vi "Write Switch Heater (No Objects).vi"(8 "error in (no error)":errorcluster, 10 "Turn SH On?":bool, 11 "Cluster In":T4={"Field"=0.0, "Rate"=0.0, "Status"={"Sweeping"=FALSE, "Clamped"=FALSE, "Hold"=FALSE, "At Rest"=FALSE, "Quench"=FALSE, "Persistent Mode"=FALSE, "Switch Heater"=FALSE}, "ILM Shut Down?"=FALSE, "IO Info"={"Address"={"Com Port"=1, "ISOBUS Address"=2, "GPIB Address"=24, "Communication"=enum."ISOBUS"}, "Version"=enum."IPS"}, "IO Info (Level Meter)"={"Address"={"Com Port"=1, "ISOBUS Address"=5, "GPIB Address"=24, "Communication"=enum."ISOBUS"}, "ILM Name"="", "Display Channel"=[]}, "Training?"=FALSE, "Training Field and Speed Cluster"={"Training Field"=[0.0, 4.108, 5.78, 8.001], "Training Speed"=[0.0057, 0.0022833333333333334, 0.0011333333333333334, 0.0011333333333333334]}}) -> (0 "error out":errorcluster, 3 "Cluster Out":T4={"Field"=0.0, "Rate"=0.0, "Status"={"Sweeping"=FALSE, "Clamped"=FALSE, "Hold"=FALSE, "At Rest"=FALSE, "Quench"=FALSE, "Persistent Mode"=FALSE, "Switch Heater"=FALSE}, "ILM Shut Down?"=FALSE, "IO Info"={"Address"={"Com Port"=1, "ISOBUS Address"=2, "GPIB Address"=24, "Communication"=enum."ISOBUS"}, "Version"=enum."IPS"}, "IO Info (Level Meter)"={"Address"={"Com Port"=1, "ISOBUS Address"=5, "GPIB Address"=24, "Communication"=enum."ISOBUS"}, "ILM Name"="", "Display Channel"=[]}, "Training?"=FALSE, "Training Field and Speed Cluster"={"Training Field"=[0.0, 4.108, 5.78, 8.001], "Training Speed"=[0.0057, 0.0022833333333333334, 0.0011333333333333334, 0.0011333333333333334]}})   [LabVIEW 2012]
uses:
  Magnet status.ctl
  Oxford/PSSUBS.LLB/PSIO.ctl
  Oxford/BUSGEN.LLB/OxfordAddress.ctl
  Switch Heater Status.ctl
  Power Supply.lvclass
panel:
  out "true interrupt":bool
  in  "interrupt":bool
  out "done":bool
  out "busybar":bool[](array[boolean])
  out "time":string
  out "display":string
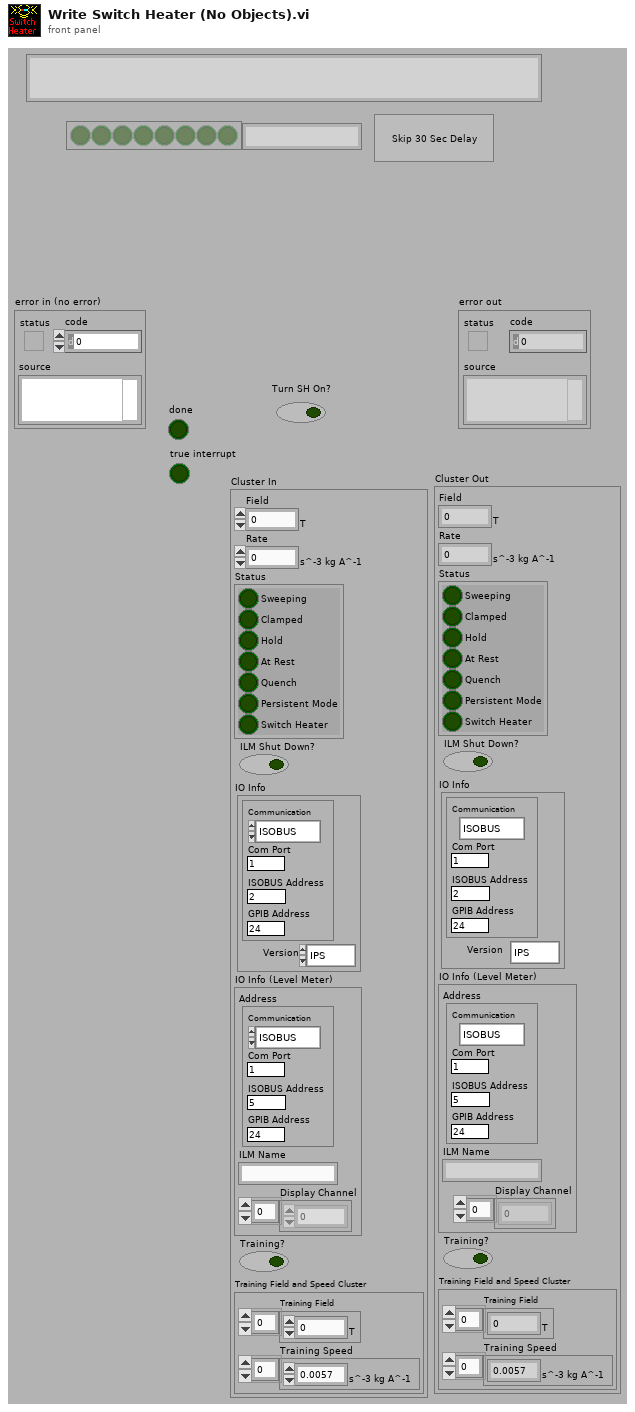
[diagram p1: front panel]
types:
  T1 = typedef "Power Supply.lvclass/Magnet status.ctl" = cluster{"Sweeping":bool, "Clamped":bool, "Hold":bool, "At Rest":bool, "Quench":bool, "Persistent Mode":bool, "Switch Heater":bool}
  T2 = typedef "PSIO.ctl" = cluster{"Address":T3, "Version":enum16{"PS", "IPS"}}
  T3 = typedef "OxfordAddress.ctl" = cluster{"Com Port":i32, "ISOBUS Address":i32, "GPIB Address":i16, "Communication":enum16{"RS232", "ISOBUS", "GPIB", "Gateway"}}
  T4 = cluster{"Field":dbl[unit], "Rate":dbl[unit], "Status":T1, "ILM Shut Down?":bool, "IO Info":T2, "IO Info (Level Meter)":cluster{"Address":T3, "ILM Name":string, "Display Channel":i32[]}, "Training?":bool, "Training Field and Speed Cluster":cluster{"Training Field":dbl[unit][], "Training Speed":dbl[unit][]}}
  T5 = typedef "Power Supply.lvclass/Switch Heater Status.ctl" = enum16{"Off (at zero)", "On", "Off (at field)", "Other"}
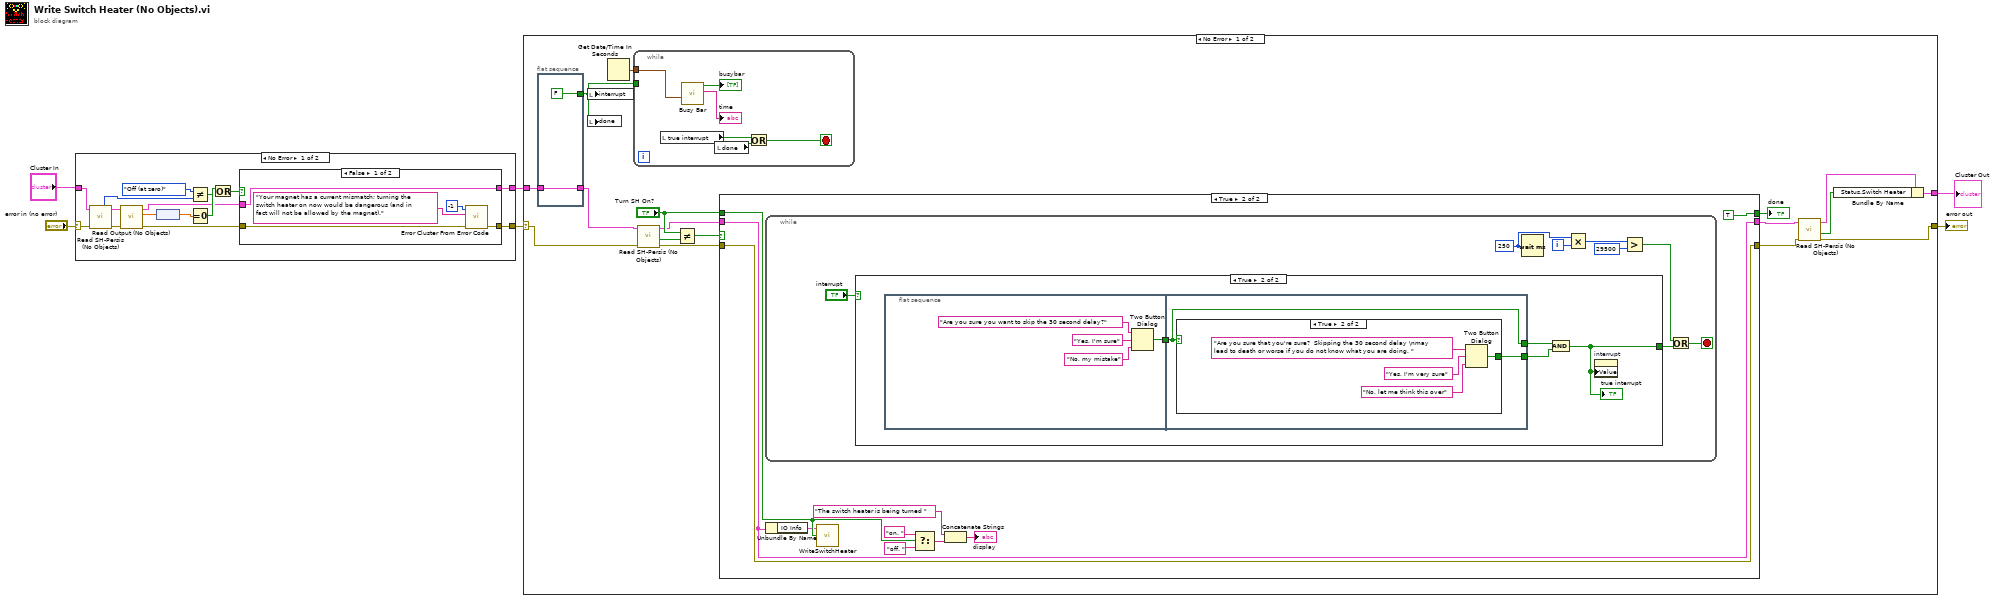
[diagram p0: block diagram]
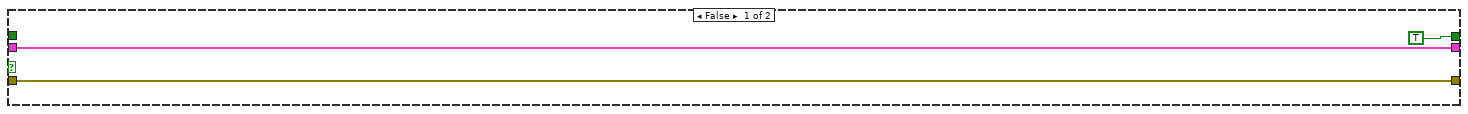
[diagram p4: hidden frame]
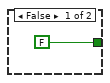
[diagram p5: hidden frame]
diagram:
  n1 = case shown="No Error" "error in (no error)" {
    selector: "error in (no error)" -> [w12 w29]
    tunnel: [w14 w30] -> w5
    tunnel: [w13 w29] -> w4
    tunnel: "Cluster In" -> [w8 w30]
    frame No Error {
      n2 = call "Read SH-Persis (No Objects).vi"("error in (no error)"=w12, "Cluster In"=w8) -> ("error out"=w17:errorcluster, "Cluster Out"=w7:T4, "SHstatus"=w11:T5)  [unwired: 4 in, 3 out]
      n3 = call "Read Output (No Objects).vi"("error in (no error)"=w17, "Cluster In"=w7) -> ("error out"=w18:errorcluster, "Field"=w19:dbl[unit], "Cluster Out"=w16:T4)  [unwired: 6 in, 1 out]
      n4 = node(w19) -> (w15:dbl)
      n5 = Not Equal?(x=Switch_Heater_Status."Off (at zero)", y=w11) -> (x != y?=w9:bool)
      n6 = Equal To 0?(x=w15) -> (x = 0?=w21:bool)
      n7 = Or(x=w21, y=w9) -> (x .or. y?=w20:bool)
      n8 = case shown="False" w20 {
        tunnel: w18 -> [w25 w28]
        tunnel: w16 -> [w26 w27]
        tunnel: [w26 w27] -> w14
        tunnel: [w24 w28] -> w13
        frame False {
          n9 = call <vilib>:"Error Cluster From Error Code.vi"("error in (no error)"=w25, "error message (\"\")"="Your magnet has a current mismatch; turning the switch heater on now would be dangerous (and in fact will not be allowed by the magnet).", "error code (0)"=-1) -> ("error out"=w24:errorcluster)  [unwired: 6 in]
        }
        frame True {
        }
      }
    }
    frame Error {
    }
  }
  n10 = case shown="No Error" w4 {
    selector: w4 -> [w44 w92]
    tunnel: w5 -> [w47 w93]
    tunnel: [w46 w93] -> w1
    tunnel: [w45 w92] -> w6
    frame No Error {
      n11 = flat-sequence {
        tunnel: w47 -> [w91]
        tunnel: [w91] -> w32
        tunnel: [FALSE] -> w33
        frame #0 {
        }
      }
      n12 = local write "interrupt"(w33) -> ()
      n13 = local write "done"(w33) -> ()
      n14 = Get Date/Time In Seconds() -> (seconds since 1Jan1904=w43:timestamp)
      n15 = while {
        tunnel: w43 -> [w84]
        tunnel: w33 -> [_]
        stop <- w87 stop-if-true
        n16 = local read "true interrupt"() -> (w85:bool)
        n17 = call "Busy Bar.vi"("basetime"=w84) -> ("Time"=→"time":string, "Busy Bar"=→"busybar":bool[])  [unwired: 1 in, 8 out]
        n18 = local read "done"() -> (w86:bool)
        n19 = Or(x=w85, y=w86) -> (x .or. y?=w87:bool)
      }
      n20 = call "Read SH-Persis (No Objects).vi"("error in (no error)"=w44, "Cluster In"=w32) -> ("error out"=w37:errorcluster, "SHon?"=w39:bool, "Cluster Out"=w38:T4)  [unwired: 4 in, 3 out]
      n21 = Not Equal?(x="Turn SH On?", y=w39) -> (x != y?=w41:bool)
      n22 = case shown="True" w41 {
        tunnel: "Turn SH On?" -> [_ w60]
        tunnel: [w50 w54] -> w31
        tunnel: w38 -> [w50 w54]
        tunnel: w37 -> [w49 w52]
        tunnel: [w49 w52] -> w42
        tunnel: [TRUE TRUE] -> w36
        frame False {
        }
        frame True {
          n23 = while {
            i -> [w67]
            stop <- w68 stop-if-true
            w66 = 250
            n24 = case shown="True" "interrupt" {
              tunnel: [FALSE w70] -> w61
              frame False {
              }
              frame True {
                n25 = flat-sequence {
                  tunnel: [w74] -> w71
                  tunnel: [w78] -> w73
                  tunnel: w71 -> [w78]
                  tunnel: [w79] -> w72
                  frame #0 {
                    n26 = Two Button Dialog(message="Are you sure you want to skip the 30 second delay?", 1:"No, my mistake", 2:"Yes, I'm sure") -> (T button?=w74:bool)
                  }
                  frame #1 {
                    n27 = case shown="True" w78 {
                      tunnel: [_ w80] -> w79
                      frame False {
                      }
                      frame True {
                        n28 = Two Button Dialog(message="Are you sure that you're sure?  Skipping the 30 second delay \nmay lead to death or worse if you do not know what you are doing. ", 1:"No, let me think this over", 2:"Yes, I'm very sure") -> (T button?=w80:bool)
                      }
                    }
                  }
                }
                n29 = And(x=w73, y=w72) -> (x .and. y?=w70:bool)
                "true interrupt" <- w70
                n30 = property on="interrupt" class="Bool (strict)"("Value"=w70) -> ()  [unwired: 2 in, 2 out]
              }
            }
            n31 = Wait (ms)(milliseconds to wait=w66) -> ()  [unwired: 1 out]
            n32 = Multiply(x=w66, y=w67) -> (x*y=w65:i32)
            n33 = Greater?(x=w65, y=29500) -> (0:w64:bool)
            n34 = Or(x=w64, y=w61) -> (x .or. y?=w68:bool)
          }
          n35 = Unbundle By Name(w54) -> ("IO Info"=w53:T2)
          n36 = call "WriteSwitchHeater.vi"("Switch Heater On"=w60, "IO Info"=w53) -> ()  [unwired: 1 in, 2 out]
          n37 = Select(t="on. ", s=w60, f="off. ") -> (s? t:f=w56:string)
          n38 = Concatenate Strings("The switch heater is being turned ", w56) -> (→"display":string)
        }
      }
      "done" <- w36
      n39 = call "Read SH-Persis (No Objects).vi"("error in (no error)"=w42, "Cluster In"=w31) -> ("error out"=w45:errorcluster, "SHon?"=w34:bool, "Cluster Out"=w35:T4)  [unwired: 4 in, 3 out]
      n40 = Bundle By Name(cluster=w35, "Status.Switch Heater"=w34) -> (w46:T4)
    }
    frame Error {
    }
  }
  "error out" <- w6
  "Cluster Out" <- w1
